vi "MultiplicationUI.vi"(0 "Multiply in":refnum<class "Multiply.lvclass">, 1 "B":dbl, 5 "A":dbl, 7 "user event out":refnum<user-event>, 9 "event source":refnum<user-event>, 11 "error in (no error)":errorcluster, 12 "Calculate":bool) -> (4 "Multiply out":refnum<class "Multiply.lvclass">, 6 "C":dbl, 15 "error out":errorcluster)   [LabVIEW 2023, in "Multiply.lvclass"]
uses:
  Multiply.lvclass
  C:/Users/santharu.subramanian/Documents/LV New Assignments/DVR in OOPS/Classes/Arithmetic/Arithmetic.lvclass
  Arithmetic/Arithmetic.lvclass
  Multiply.lvclass/Multiply.ctl
panel:
  # "MULTIPLICATION"
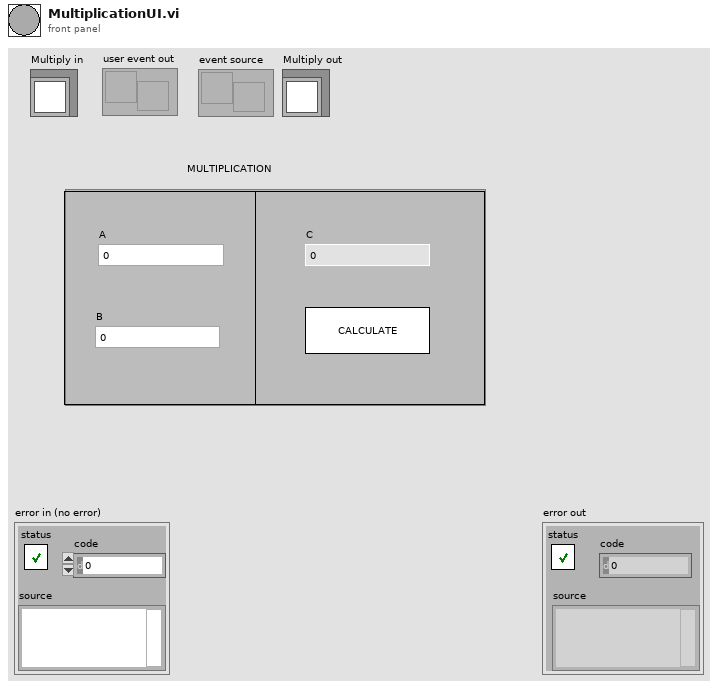
[diagram p1: front panel]
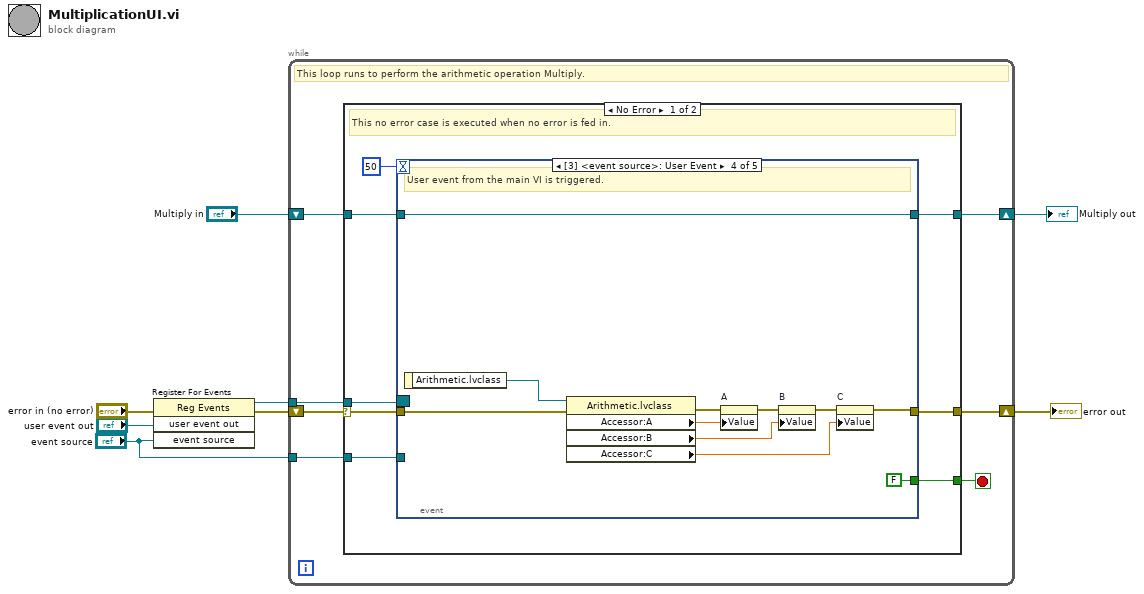
[diagram p0: block diagram]
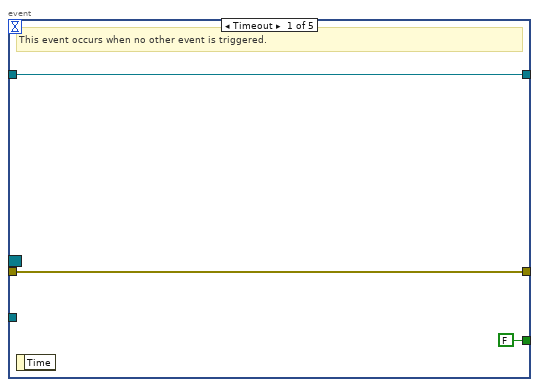
[diagram p2: hidden frame]
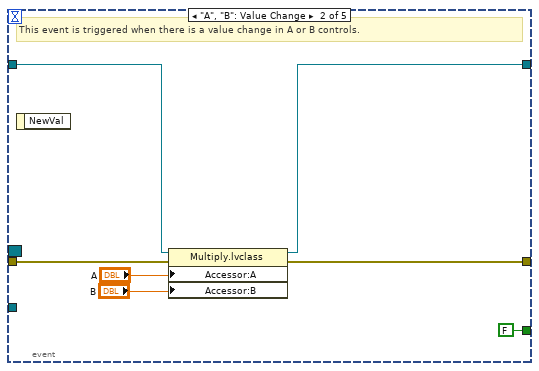
[diagram p3: hidden frame]
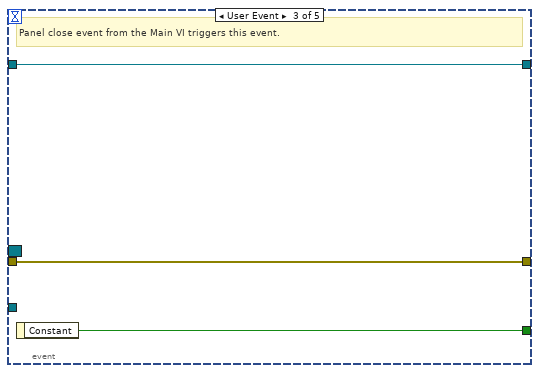
[diagram p4: hidden frame]
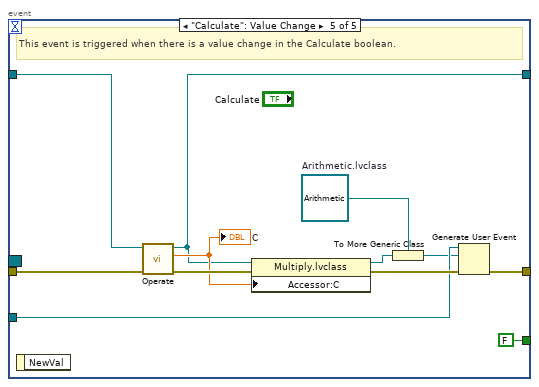
[diagram p5: hidden frame]
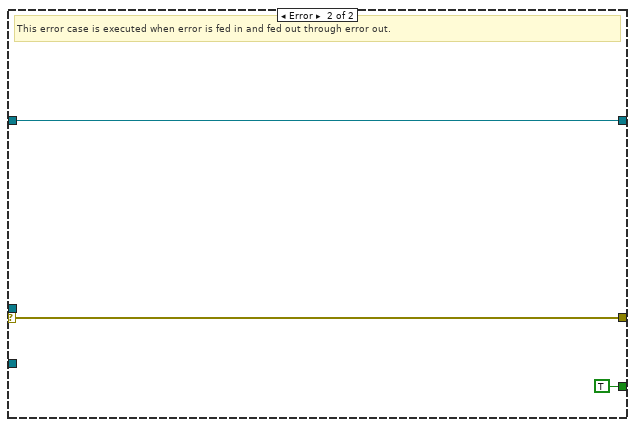
[diagram p6: hidden frame]
diagram:
  n1 = register-events(error in="error in (no error)", "user event out", "event source") -> (reference out=w2:refnum<event-registration>, error out=w3:errorcluster)  [unwired: 1 in]
  n2 = while {
    shift-right: [w14] -> w6
    shift-left: w3 -> [w15]
    shift-right: [w12] -> w7
    shift-left: "Multiply in" -> [w13]
    tunnel: w2 -> [w11]
    tunnel: "event source" -> [w9]
    stop <- w10 stop-if-true
    # "This loop runs to perform the arithmetic operation Multiply."
    n3 = case shown="No Error" w15 {
      selector: w15 -> [w23 w62]
      tunnel: [w22 w62] -> w14
      tunnel: [w20 w61] -> w12
      tunnel: w13 -> [w21 w61]
      tunnel: w11 -> [w18 _]
      tunnel: [w17 TRUE ("Constant")] -> w10
      tunnel: w9 -> [w16 _]
      frame No Error {
        # "This no error case is executed when no error is fed in."
        n4 = event shown="[3] <event source>: User Event" {
          selector: w18 -> [_ _ _ _ _]
          dyn-events: _ -> [_ _ _ _ _]
          timeout: 50 -> [_ _ _ _ _]
          tunnel: w23 -> [w26 w32 w35 w45 w59]
          tunnel: [w26 w31 w35 w46 w54] -> w22
          tunnel: w21 -> [w25 w33 w36 w47 w51]
          tunnel: [w25 w28 w36 w47 w50] -> w20
          tunnel: [FALSE ("Constant") FALSE ("Constant") w34 FALSE ("Constant") FALSE ("Constant")] -> w17
          tunnel: w16 -> [_ _ _ _ w52]
          event Timeout {
            # "This event occurs when no other event is triggered."
            n5 = event-data() -> ()  [unwired: 1 in, 1 out]
          }
          event "A", "B": Value Change {
            # "This event is triggered when there is a value change in A or B controls."
            n6 = event-data() -> ()  [unwired: 1 in, 1 out]
            n7 = property class="Multiply.lvclass"(reference=w33, error in=w32, "Accessor:A"="A", "Accessor:B"="B") -> (reference out=w28:refnum<class "Multiply.lvclass">, error out=w31:errorcluster)
          }
          event User Event {
            # "Panel close event from the Main VI triggers this event."
            n8 = event-data() -> ("Constant"=w34:bool)  [unwired: 1 in]
          }
          event User Event {
            # "User event from the main VI is triggered."
            n9 = event-data() -> ("Arithmetic.lvclass"=w44:refnum<class "Arithmetic.lvclass">)  [unwired: 1 in]
            n10 = property class="Arithmetic.lvclass"(reference=w44, error in=w45) -> (error out=w42:errorcluster, "Accessor:A"=w41:dbl, "Accessor:B"=w38:dbl, "Accessor:C"=w37:dbl)  [unwired: 1 out]
            n11 = property on="A" class="DigNum (strict)"(error in=w42, "Value"=w41) -> (error out=w40:errorcluster)  [unwired: 1 in, 1 out]
            n12 = property on="B" class="DigNum (strict)"(error in=w40, "Value"=w38) -> (error out=w39:errorcluster)  [unwired: 1 in, 1 out]
            n13 = property on="C" class="DigNum (strict)"(error in=w39, "Value"=w37) -> (error out=w46:errorcluster)  [unwired: 1 in, 1 out]
          }
          event "Calculate": Value Change {
            w49 = refnum<class "Arithmetic.lvclass"> refnum  # Arithmetic.lvclass
            # "This event is triggered when there is a value change in the Calculate boolean."
            n14 = event-data() -> ()  [unwired: 1 in, 1 out]
            n15 = call-dynamic "Operate.vi"("error in (no error)"=w59, "Multiply in"=w51) -> ("error out"=w55:errorcluster, "C"=w53:dbl, "Multiply out"=w50:refnum<class "Multiply.lvclass">)  [unwired: 7 in]
            "C" <- w53
            n16 = property class="Multiply.lvclass"(reference=w50, error in=w55, "Accessor:C"=w53) -> (reference out=w56:refnum<class "Multiply.lvclass">, error out=w57:errorcluster)
            n17 = To More Generic Class(target class=w49, reference=w56) -> (generic class reference=w48:refnum<class "Arithmetic.lvclass">)
            n18 = Generate User Event(user event=w52, event data cluster=w48, error in=w57) -> (error out=w54:errorcluster)  [unwired: 1 in, 1 out]
          }
        }
      }
      frame Error {
        # "This error case is executed when error is fed in and fed out through error out."
      }
    }
  }
  "error out" <- w6
  "Multiply out" <- w7
